vi "writeU16FIFO.vi"(8 "error in (no error)":errorcluster, 9 "Timeout":i32, 10 "Data":u16[](array[numeric]), 11 "ModbusSubnetATxDataFIFO in":refnum<class "ModbusSubnetATxDataFIFO.lvclass">) -> (0 "error out":errorcluster, 2 "ElementsRemaining":u32, 3 "ModbusSubnetATxDataFIFO out":refnum<class "ModbusSubnetATxDataFIFO.lvclass">)   [LabVIEW 2016, in "ModbusSubnetATxDataFIFO.lvclass"]
uses:
  ModbusSubnetATxDataFIFO.lvclass
  ModbusSubnetATxDataFIFO.lvclass/ModbusSubnetATxDataFIFO.ctl
  FPGA/FPGA.lvclass
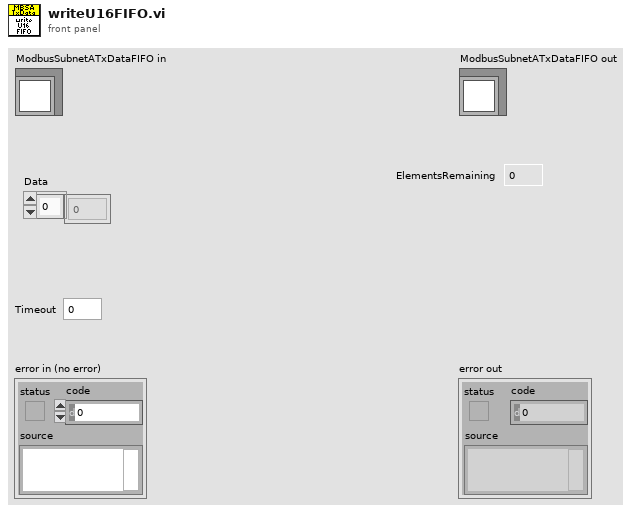
[diagram p1: front panel]
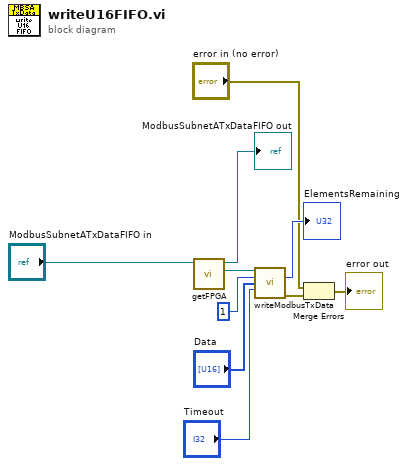
[diagram p0: block diagram]
diagram:
  n1 = call "getFPGA.vi"("ModbusSubnetATxDataFIFO in"="ModbusSubnetATxDataFIFO in") -> ("FPGA"=w8:refnum<class "FPGA.lvclass">, "ModbusSubnetATxDataFIFO out"=→"ModbusSubnetATxDataFIFO out":refnum<class "ModbusSubnetATxDataFIFO.lvclass">)  [unwired: 9 in]
  n2 = call "writeModbusTxData.vi"("FPGA in"=w8, "Subnet"=u16 1, "Data"="Data", "Timeout (ms)"="Timeout") -> ("Empty Elements Remaining"=→"ElementsRemaining":u32, "error out"=w3:errorcluster)  [unwired: 9 in, 1 out]
  n3 = Merge Errors("error in (no error)", w3) -> (→"error out":errorcluster)
